vi "7 Segment Dispaly.vi"(11 "Ring":u16) -> (0 "D":bool, 1 "G":bool, 2 "F":bool, 3 "C":bool, 4 "E":bool, 5 "B":bool, 6 "DP":bool, 7 "A":bool)   [LabVIEW 2018]
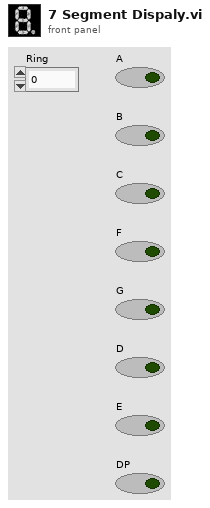
[diagram p1: front panel]
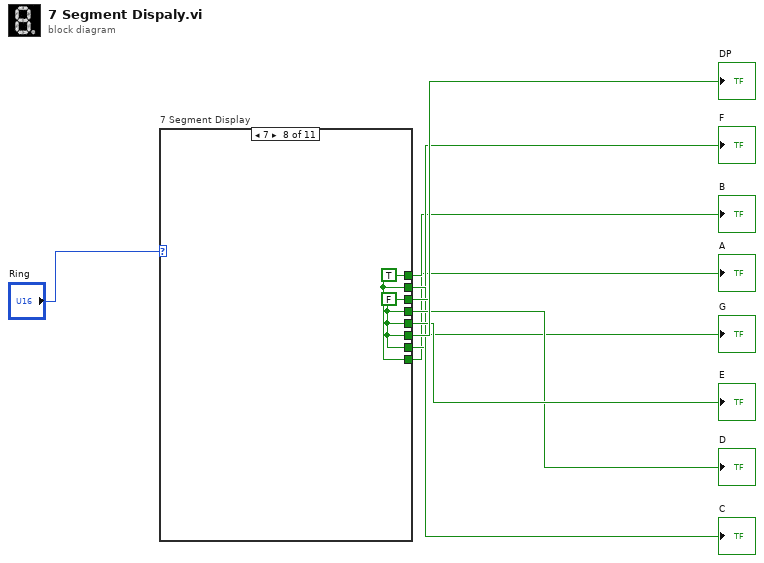
[diagram p0: block diagram]
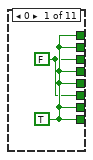
[diagram p2: hidden frame]
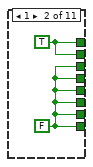
[diagram p3: hidden frame]
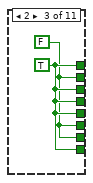
[diagram p4: hidden frame]
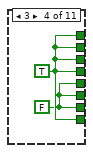
[diagram p5: hidden frame]
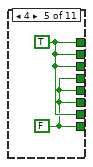
[diagram p6: hidden frame]
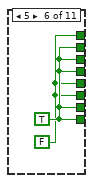
[diagram p7: hidden frame]
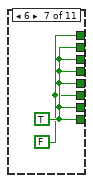
[diagram p8: hidden frame]
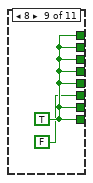
[diagram p9: hidden frame]
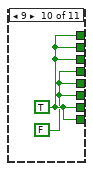
[diagram p10: hidden frame]
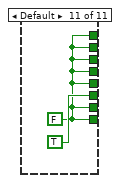
[diagram p11: hidden frame]
diagram:
  n1 = case "7 Segment Display" shown="7" "Ring" {
    tunnel: [w11 w12 w15 w17 w18 w21 w23 w25 w27 w29 w30] -> w1
    tunnel: [w11 w13 w15 w17 w19 w20 w22 w25 w27 w29 w30] -> w2
    tunnel: [w11 w12 w14 w16 w19 w21 w23 w24 w27 w29 w30] -> w3
    tunnel: [w11 w13 w14 w17 w19 w21 w23 w25 w27 w29 w30] -> w4
    tunnel: [w10 w12 w15 w17 w19 w21 w23 w24 w27 w29 w30] -> w5
    tunnel: [w11 w12 w15 w17 w18 w21 w23 w24 w27 w28 w30] -> w6
    tunnel: [w11 w12 w15 w16 w18 w20 w23 w24 w27 w28 w30] -> w7
    tunnel: [w10 w12 w14 w16 w18 w20 w22 w24 FALSE w28 TRUE] -> w8
    frame 0 {
      w10 = FALSE
      w11 = TRUE
    }
    frame 1 {
      w12 = FALSE
      w13 = TRUE
    }
    frame 2 {
      w14 = FALSE
      w15 = TRUE
    }
    frame 3 {
      w16 = FALSE
      w17 = TRUE
    }
    frame 4 {
      w18 = FALSE
      w19 = TRUE
    }
    frame 5 {
      w20 = FALSE
      w21 = TRUE
    }
    frame 6 {
      w22 = FALSE
      w23 = TRUE
    }
    frame 7 {
      w24 = FALSE
      w25 = TRUE
    }
    frame 8 {
      w27 = TRUE
    }
    frame 9 {
      w28 = FALSE
      w29 = TRUE
    }
    frame Default {
      w30 = FALSE
    }
  }
  "DP" <- w8
  "E" <- w7
  "D" <- w6
  "G" <- w5
  "C" <- w4
  "F" <- w3
  "B" <- w2
  "A" <- w1
